vi "Periodic Tasks.vi"(8 "error in":errorcluster) -> ()   [LabVIEW 2017]
doc: "This VI runs in parallel to other tasks. It can contain as many user-defined periodic loops as you need. These can carry out PID or other sorts of timed response."
uses:
  <vilib>/Rock Robotics/WPI/Solenoid/WPI_SolenoidValue.ctl
  <vilib>/Rock Robotics/WPI/Utilities/WPI_GetSetVariantRefNum.vi
  <vilib>/Rock Robotics/WPI/Solenoid/WPI_SolenoidSetEnum.vi
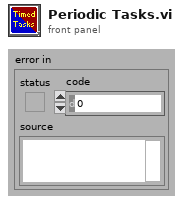
[diagram p1: front panel]
types:
  T1 = typedef "WPI_JoystickDevRef.ctl" = cluster{"Device":T2}
  T2 = typedef "WPI_JoystickDeviceEnum.ctl" = enum16{"USB 0", "USB 1", "USB 2", "USB 3", "USB 4", "USB 5"}
  T3 = typedef "WPI_RobotDriveDevRef.ctl" = cluster{"DevStatus":errorcluster, "Motors[]":T4[], "Square Inputs":bool, "Max Output":dbl}
  T4 = typedef "WPI_MotorControlDeviceRef.ctl" = cluster{"DeviceStatus":errorcluster, "Type":T5, "PWM":cluster{"PWM Channel":T6, "DeadBand":T7}, "CAN":cluster{"Device Number":u8, "SetOutput VI Ref":variant, "GetOutput VI Ref":variant, "Enable VI Ref":variant, "Disable VI Ref":variant, "Data":variant}, "Invert":bool, "DIO PWM":cluster{"PWM \"Enable\" Channel":T6, "DIOChannel":T8, "PWM Rate":dbl}}
  T5 = typedef "WPI_MotorControlType.ctl" = enum16{"PWM", "CAN", "DIO PWM"}
  T6 = typedef "FPGA_DIOPWMChannel.ctl" = enum8{"PWM 0", "PWM 1", "PWM 2", "PWM 3", "PWM 4", "PWM 5", "PWM 6", "PWM 7", "PWM 8", "PWM 9", "PWM MXP 0", "PWM MXP 1", "PWM MXP 2", "PWM MXP 3", "PWM MXP 4", "PWM MXP 5", "PWM MXP 6", "PWM MXP 7", "PWM MXP 8", "PWM MXP 9", "Invalid"}
  T7 = typedef "WPI_PWMDeadband.ctl" = cluster{"Name":string, "maxPositivePwm":i32, "minPositivePwm":i32, "centerPwm":i32, "maxNegativePwm":i32, "minNegativePwm":i32, "angularRange":u16}
  T8 = typedef "FPGA_DIOChannel.ctl" = enum8{"DIO 0", "DIO 1", "DIO 2", "DIO 3", "DIO 4", "DIO 5", "DIO 6", "DIO 7", "DIO 8", "DIO 9", "DIO MXP 0", "DIO MXP 1", "DIO MXP 2", "DIO MXP 3", "DIO MXP 4", "DIO MXP 5", "DIO MXP 6", "DIO MXP 7", "DIO MXP 8", "DIO MXP 9", "DIO MXP 10", "DIO MXP 11", "DIO MXP 12", "DIO MXP 13", "DIO MXP 14", "DIO MXP 15", "SPI Port CS1", "SPI Port CS2", "SPI Port CS3", "SPI Port MISO", "SPI Port MOSI", "Invalid"}
  T9 = typedef "WPI_ServoDeviceRef.ctl" = cluster{"DeviceStatus":errorcluster, "PWM Channel":T6, "DeadBand":T7}
  T10 = cluster{"JoystickDevRef":T1, "RobotDriveDevRef":T3, "ServoDeviceRef":T9}
  T11 = typedef "WPI_SolenoidValue.ctl" = enum16{"Off", "On", "Forward", "Reverse"}
  T12 = cluster{"Axes[0]":dbl, "Axes[1]":dbl, "Axes[2]":dbl, "Axes[3]":dbl, "Axes[4]":dbl, "Axes[5]":dbl, "Axes[6]":dbl, "Axes[7]":dbl, "Axes[8]":dbl}
  T13 = cluster{"Buttons[0]":bool, "Buttons[1]":bool, "Buttons[2]":bool, "Buttons[3]":bool, "Buttons[4]":bool, "Buttons[5]":bool, "Buttons[6]":bool, "Buttons[7]":bool, "Buttons[8]":bool}
  T14 = typedef "WPI_SolenoidDevRef.ctl" = cluster{"DevStatus":errorcluster, "Pneumatics Control Module":u8, "Forward Solenoid Channel":T15, "Reverse Solenoid Channel":T15}
  T15 = typedef "WPI_SolenoidChannel.ctl" = enum8{"Solenoid 0", "Solenoid 1", "Solenoid 2", "Solenoid 3", "Solenoid 4", "Solenoid 5", "Solenoid 6", "Solenoid 7", "Invalid"}
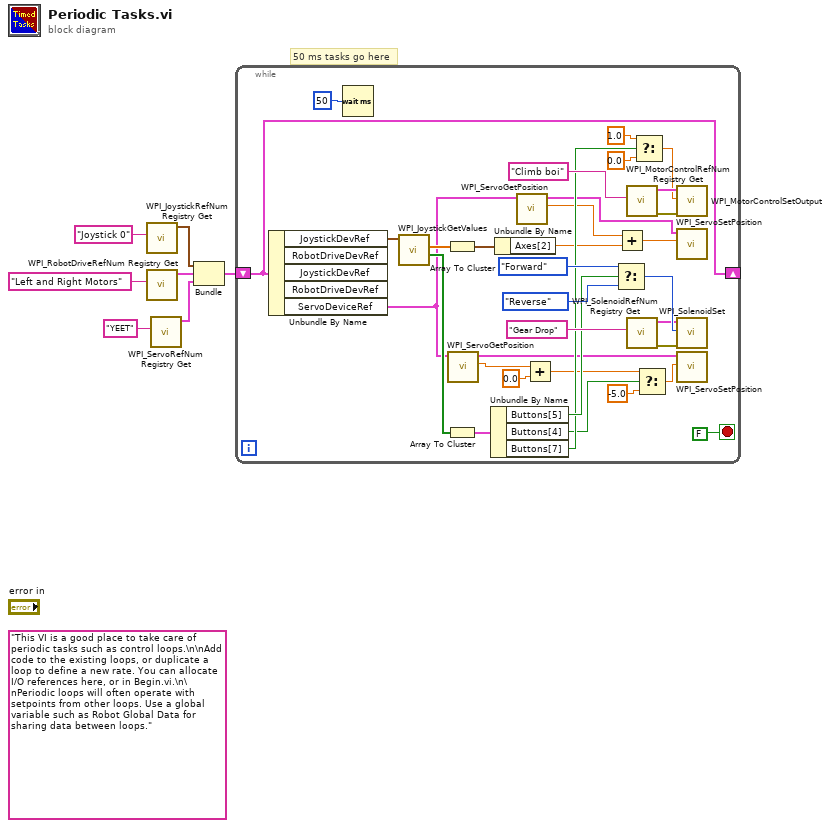
[diagram p0: block diagram]
diagram:
  (unwired) "This VI is a good place to take care of periodic tasks such as control loops.\n\nAdd code to the existing loops, or duplicate a loop to define a new rate. You can allocate I/O references here, or in Begin.vi.\n\nPeriodic loops will often operate with setpoints from other loops. Use a global variable such as Robot Global Data for sharing data between loops."
  # "50 ms tasks go here"
  n1 = call <vilib>:"WPI_JoystickRefNum Registry Get.vi"("refnum name"="Joystick 0") -> ("JoystickDevRef"=w5:T1)  [unwired: 1 in, 9 out]
  n2 = call <vilib>:"WPI_RobotDriveRefNum Registry Get.vi"("refnum name"="Left and Right Motors") -> ("RobotDriveDevRef"=w4:T3)  [unwired: 1 in, 9 out]
  n3 = call <vilib>:"WPI_ServoRefNum Registry Get.vi"("refnum name"="YEET") -> ("ServoDeviceRef"=w2:T9)  [unwired: 9 in, 1 out]
  n4 = Bundle("JoystickDevRef"=w5, "RobotDriveDevRef"=w4, "ServoDeviceRef"=w2) -> (w3:T10)  [unwired: 1 out]
  n5 = while {
    shift-right: [w39] -> _
    shift-left: w3 -> [w39]
    stop <- FALSE stop-if-true
    n6 = Unbundle By Name "Unbundle By Name"(w39) -> ("JoystickDevRef"=w38:T1, "ServoDeviceRef"=w12:T9)  [unwired: 3 out]
    n7 = Wait (ms)(milliseconds to wait=u32 50) -> ()  [unwired: 1 out]
    n8 = call <vilib>:"WPI_JoystickGetValues.vi"("JoystickDevRef"=w38) -> ("Buttons"=w33:bool[], "Axes"=w14:dbl[])  [unwired: 6 in, 3 out]
    n9 = Array To Cluster(array=w14) -> (cluster=w13:T12)
    n10 = Array To Cluster(array=w33) -> (cluster=w37:T13)
    n11 = call <vilib>:"WPI_ServoGetPosition.vi"("ServoDeviceRef"=w12) -> ("Position"=w17:dbl, "ServoDeviceRef"=w20:T9)  [unwired: 8 in, 1 out]
    n12 = Unbundle By Name(w37) -> ("Buttons[5]"=w26:bool, "Buttons[4]"=w21:bool, "Buttons[7]"=w25:bool)
    n13 = Unbundle By Name(w13) -> ("Axes[2]"=w9:dbl)
    n14 = call <vilib>:"WPI_ServoGetPosition.vi"("ServoDeviceRef"=w12) -> ("Position"=w10:dbl, "ServoDeviceRef"=w11:T9)  [unwired: 8 in, 1 out]
    n15 = Add(x=w17, y=0.0) -> (x+y=w18:dbl)
    n16 = Select(t=WPI_SolenoidValue."Forward" ("Value"), s=w26, f=WPI_SolenoidValue."Reverse" ("Value")) -> (s? t:f=w30:T11)
    n17 = Add(x=w10, y=w9) -> (x+y=w8:dbl)
    n18 = call <vilib>:"WPI_MotorControlRefNum Registry Get.vi"("refnum name"="Climb boi") -> ("error out"=w36:errorcluster, "MotorControlDevRef"=w35:T4)  [unwired: 9 in]
    n19 = call <vilib>:"WPI_SolenoidRefNum Registry Get.vi"("refnum name"="Gear Drop") -> ("error out"=w28:errorcluster, "SolenoidDevRef"=w29:T14)  [unwired: 9 in]
    n20 = Select(t=1.0, s=w25, f=0.0) -> (s? t:f=w22:dbl)
    n21 = Select(t=w18, s=w21, f=-5.0) -> (s? t:f=w19:dbl)
    n22 = call <vilib>:"WPI_MotorControlSetOutput.vi"("error in (no error)"=w36, "Output"=w22, "MotorControlDevRef"=w35) -> ()  [unwired: 6 in, 3 out]
    n23 = call <vilib>:"WPI_ServoSetPosition.vi"("Position"=w8, "ServoDeviceRef"=w11) -> ()  [unwired: 8 in, 2 out]
    n24 = call-poly <vilib>:"WPI_SolenoidSet.vi"("error in (no error)"=w28, "Value"=w30, "SolenoidDevRef"=w29) -> ()  [unwired: 7 in, 2 out]
    n25 = call <vilib>:"WPI_ServoSetPosition.vi"("Position"=w19, "ServoDeviceRef"=w20) -> ()  [unwired: 8 in, 2 out]
  }
